vi "ConfigureHardware.vi"(8 "error in (no error)":errorcluster, 11 "DAQ Hardware In":T1={"Task"="", "Max"=5.0, "min"=-5.0, "Samples Rate"=1000.0, "Channels"=[]} {"min" format="%0.2f"; "Max" format="%0.2f"}) -> (0 "error out":errorcluster, 3 "DAQ Hardware Out":T1={"Task"="", "Max"=5.0, "min"=-5.0, "Samples Rate"=1000.0, "Channels"=[]} {"min" format="%0.2f"; "Max" format="%0.2f"})   [LabVIEW 2014, in "NIDAQ.lvlib"]
uses:
  NIDAQ.lvlib
  DAQHardware.ctl
  <vilib>/DAQmx/create/channels.llb/DAQmx Create Channel (AI-Voltage-Basic).vi
  <vilib>/DAQmx/configure/timing.llb/DAQmx Timing (Sample Clock).vi
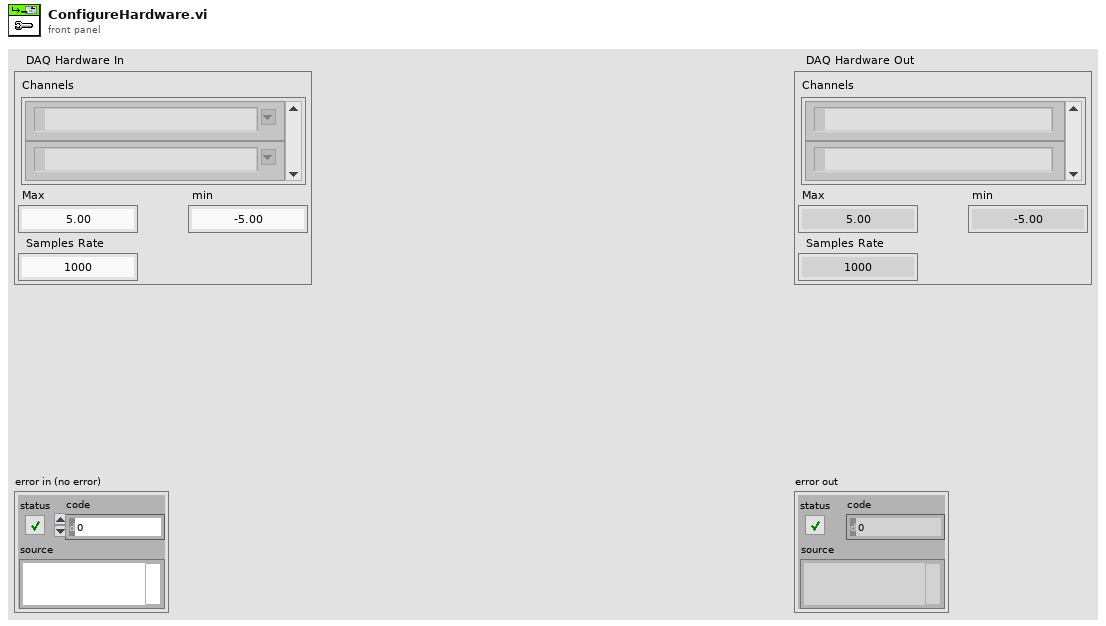
[diagram p1: front panel]
types:
  T1 = typedef "NIDAQ.lvlib/DAQHardware.ctl" = cluster{"Task":refnum<k21>, "Max":dbl, "min":dbl, "Samples Rate":dbl, "Channels":tag[]}
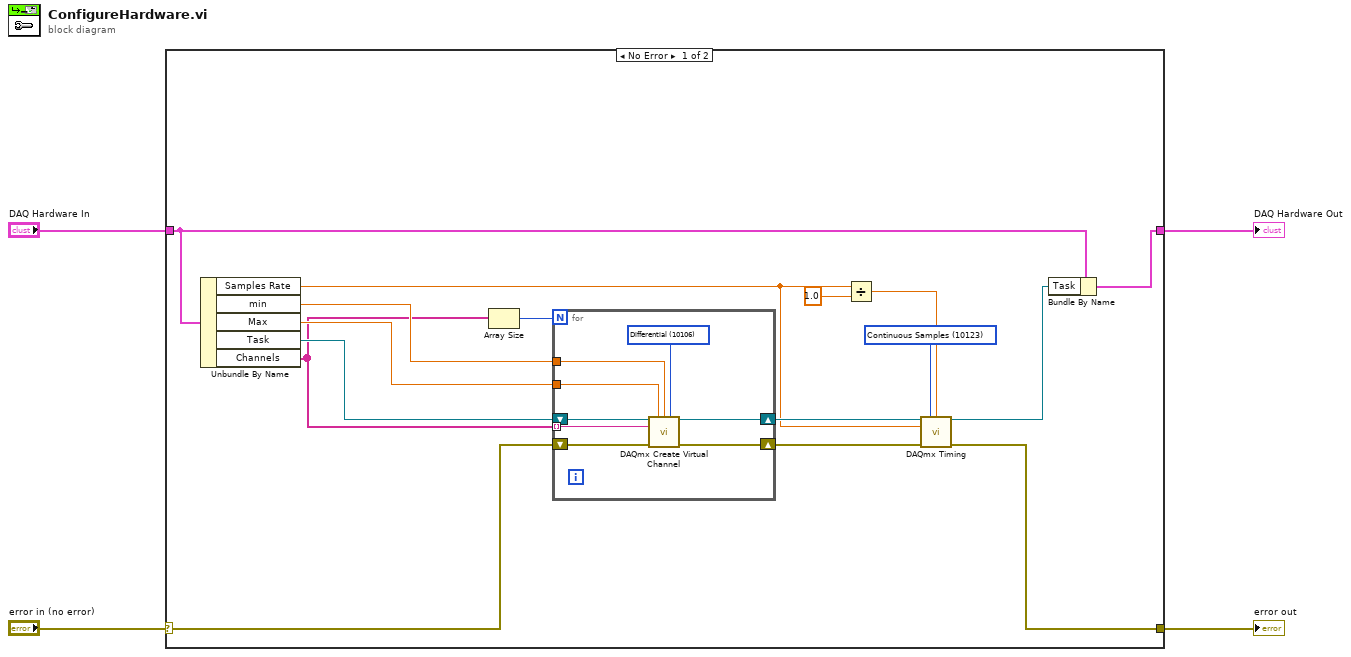
[diagram p0: block diagram]
diagram:
  n1 = case shown="No Error" "error in (no error)" {
    selector: "error in (no error)" -> [w18 w30]
    tunnel: [w11 w30] -> w3
    tunnel: "DAQ Hardware In" -> [w14 w29]
    tunnel: [w13 w29] -> w1
    frame No Error {
      w17 = 10123 items=["Finite Samples"=10178, "Continuous Samples"=10123, "Hardware Timed Single Point"=12522] ("sample mode")
      n2 = Unbundle By Name(w14) -> ("Samples Rate"=w15:dbl, "min"=w8:dbl, "Max"=w9:dbl, "Task"=w10:refnum<k21>, "Channels"=w5:tag[])
      n3 = Array Size(array=w5) -> (size(s)=w6:i32)
      n4 = for {
        N: w6 -> [_]
        tunnel: w5 -> [w25] mode=indexing
        shift-right: [w27] -> w19
        shift-left: w18 -> [w26]
        shift-right: [w28] -> w20
        shift-left: w10 -> [w24]
        tunnel: w9 -> [w22]
        tunnel: w8 -> [w21]
        w23 = 10106 items=["default"=-1, "RSE"=10083, "NRSE"=10078, "Differential"=10106, "Pseudodifferential"=12529] ("input terminal configuration")
        n5 = call-poly <vilib>:"DAQmx Create Virtual Channel.vi"("task in"=w24, "maximum value"=w22, "minimum value"=w21, "input terminal configuration"=w23, "physical channels"=w25, "error in"=w26) -> ("task out"=w28:refnum<k21>, "error out"=w27:errorcluster)  [unwired: 8 in]
      }
      n6 = Divide(x=w15, y=1.0) -> (x/y=w16:dbl)
      n7 = call-poly <vilib>:"DAQmx Timing.vi"("task/channels in"=w20, "sample mode"=w17, "samples per channel"=w16, "rate"=w15, "error in"=w19) -> ("task out"=w12:refnum<k21>, "error out"=w11:errorcluster)  [unwired: 9 in]
      n8 = Bundle By Name(cluster=w14, "Task"=w12) -> (w13:T1)
    }
    frame Error {
    }
  }
  "error out" <- w3
  "DAQ Hardware Out" <- w1
